vi "Load from History File.vi"(8 "error in (no error)":errorcluster, 11 "Data Manager in":refnum<class "Data Manager.lvclass">) -> (0 "error out":errorcluster, 2 "History":T1={"Record Headers"=["Athlete", "Team", "Type", "Date", "Distance", "Moving Time", "Elapsed Time", "Total Elevation Gain"], "All Records"=[]}, 3 "Data Manager out":refnum<class "Data Manager.lvclass">)   [LabVIEW 2020, in "Data Manager.lvclass"]
uses:
  Data Manager.lvclass
  Data Manager.lvclass/Data Manager.ctl
  Name--cluster.ctl
  Profile--cluster.ctl
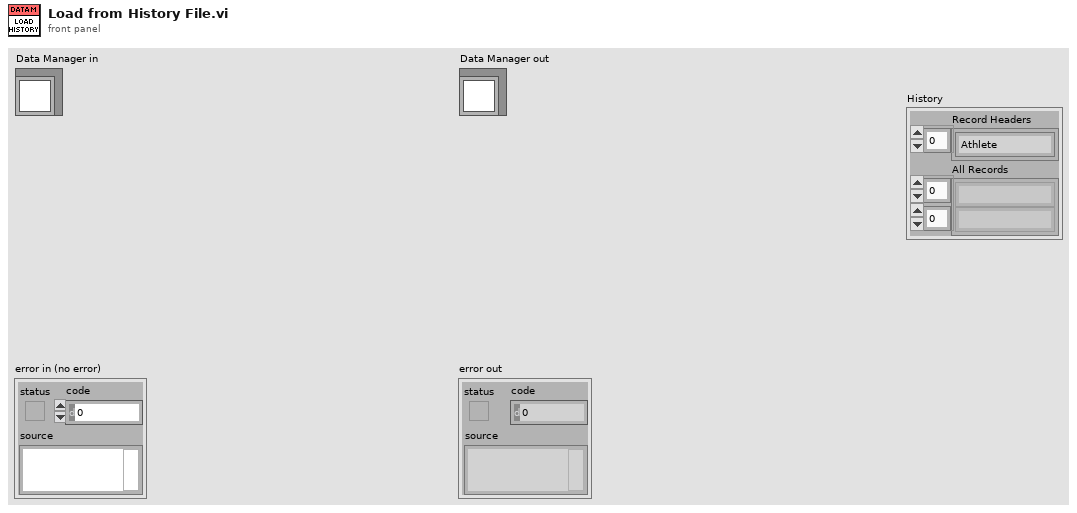
[diagram p1: front panel]
types:
  T1 = cluster{"Record Headers":string[], "All Records":string[][]}
  T2 = enum16{"open", "open or create", "create or replace", "create", "open (read-only)"}
  T3 = typedef "Data Manager.lvclass/Profile--cluster.ctl" = cluster{"Alias":string, "Team":string}
  T4 = typedef "Data Manager.lvclass/Name--cluster.ctl" = cluster{"First":string, "Last":string}
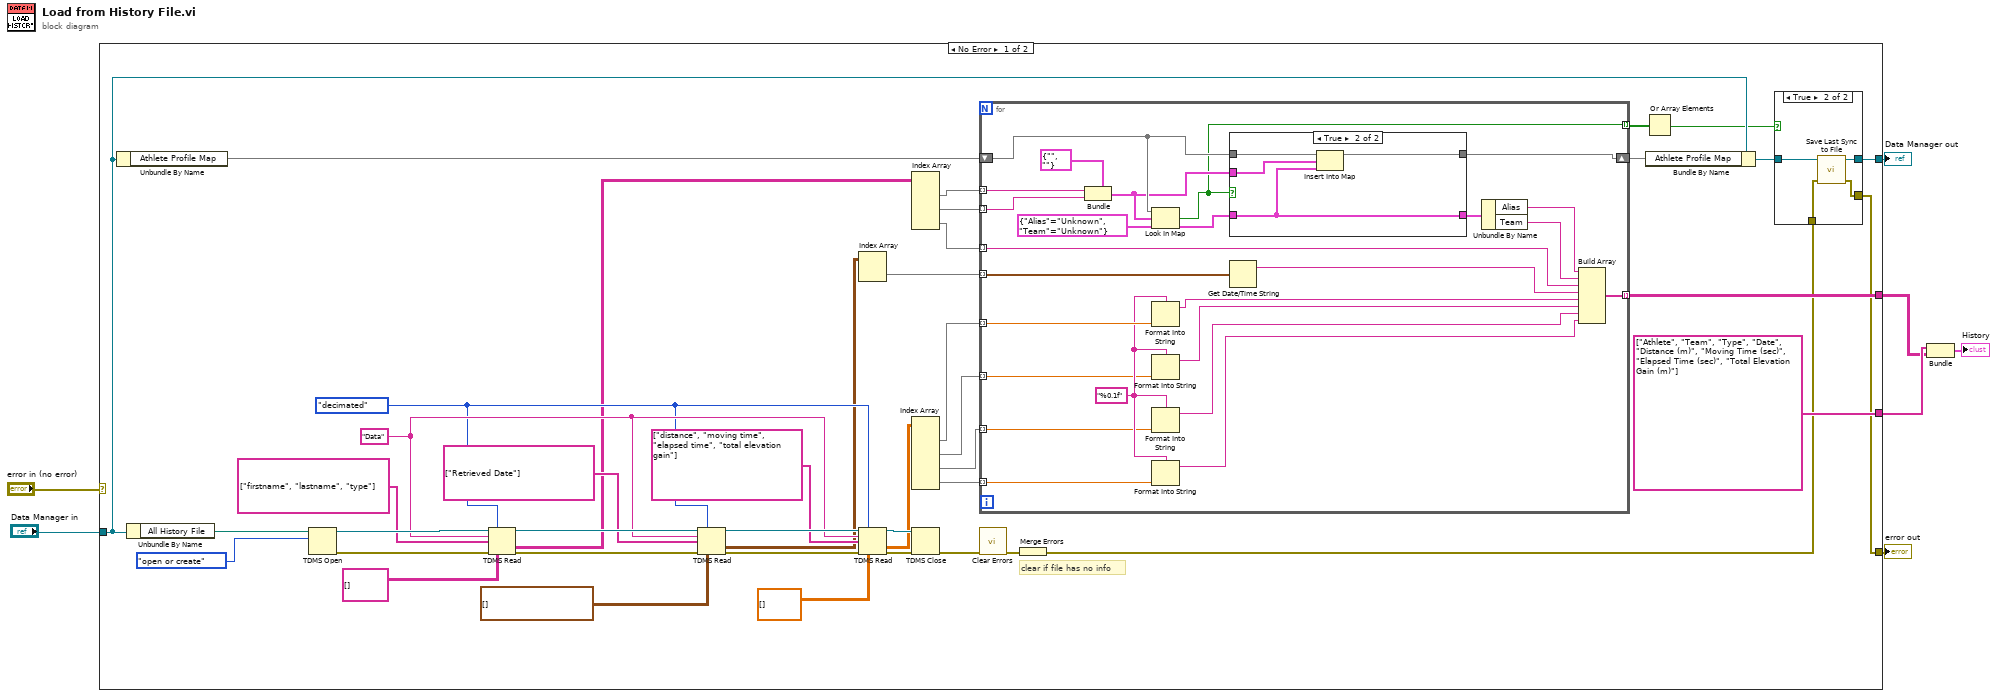
[diagram p0: block diagram]
diagram:
  n1 = case shown="No Error" "error in (no error)" {
    selector: "error in (no error)" -> [_ w88]
    tunnel: [w11 w88] -> w6
    tunnel: [w9 w87] -> w4
    tunnel: "Data Manager in" -> [w24 w87]
    tunnel: [string[] ["Athlete", "Team", "Type", "Date", "Distance (m)", "Moving Time (sec)", "Elapsed Time (sec)", "Total Elevation Gain (m)"] ("appended array") _] -> w3
    tunnel: [w15 _] -> w2
    frame No Error {
      w41 = enum16{"decimated", "interleaved"}."decimated" ("data layout (0:decimated)")
      w42 = "Data" ("group name in (Untitled)")
      # "clear if file has no info"
      n2 = Unbundle By Name(w24) -> ("Athlete Profile Map"=w26:map{T4, T3})
      n3 = Unbundle By Name(w24) -> ("All History File"=w40:path)
      n4 = TDMS Open(10:T2."open or create" ("operation (0:open)"), 11:w40) -> (0:w31:errorcluster, 3:w48:refnum<k34>)  [unwired: 5 in]
      n5 = TDMS Read(0:w48, 1:w41, 5:w42, 7:string[] ["firstname", "lastname", "type"] ("channel name(s) in (Untitled)"), 11:w31, 12:string[][] [] ("transposed array")) -> (4:w44:refnum<k34>, 10:w29:string[][], 15:w33:errorcluster)  [unwired: 2 in, 3 out]
      n6 = TDMS Read(0:w44, 1:w41, 5:w42, 7:string[] ["Retrieved Date"] ("channel name(s) in (Untitled)"), 11:w33, 12:timestamp[][] [] ("transposed array")) -> (4:w43:refnum<k34>, 10:w23:timestamp[][], 15:w32:errorcluster)  [unwired: 2 in, 3 out]
      n7 = Index Array(array=w23) -> (element=w22:timestamp[])  [unwired: 2 in]
      n8 = TDMS Read(0:w43, 1:w41, 5:w42, 7:string[] ["distance", "moving time", "elapsed time", "total elevation gain"] ("channel name(s) in (Untitled)"), 11:w32, 12:dbl[][] [] ("transposed array")) -> (4:w47:refnum<k34>, 10:w21:dbl[][], 15:w46:errorcluster)  [unwired: 2 in, 3 out]
      n9 = Index Array(array=w29) -> (element #1=w28:string[], element #2=w27:string[], element #3=w25:string[])  [unwired: 6 in]
      n10 = Index Array(array=w21) -> (element #1=w20:dbl[], element #2=w19:dbl[], element #3=w18:dbl[], element #4=w17:dbl[])  [unwired: 8 in]
      n11 = TDMS Close(8:w46, 11:w47) -> (0:w45:errorcluster)  [unwired: 1 out]
      n12 = for {
        tunnel: w28 -> [w79] mode=indexing
        tunnel: w27 -> [w78] mode=indexing
        shift-right: [w75] -> w14
        shift-left: w26 -> [w76]
        tunnel: w25 -> [w66] mode=indexing
        tunnel: w22 -> [w69] mode=indexing
        tunnel: w20 -> [w71] mode=indexing
        tunnel: w19 -> [w63] mode=indexing
        tunnel: w18 -> [w60] mode=indexing
        tunnel: w17 -> [w59] mode=indexing
        tunnel: [w57] -> w15 mode=indexing
        tunnel: [w56] -> w13 mode=indexing
        w70 = "%0.1f" ("format string")
        n13 = Bundle(cluster=T4 {"First"="", "Last"=""} ("Name"), "First"=w79, "Last"=w78) -> (w73:T4)
        n14 = Look In Map(map=w76, key=w73, default value=T3 {"Alias"="Unknown", "Team"="Unknown"}) -> (key not found?=w56:bool, value=w74:T3)
        n15 = Format Into String(format string=w70, w71) -> (resulting string=w64:string)  [unwired: 2 in, 1 out]
        n16 = Format Into String(format string=w70, w63) -> (resulting string=w62:string)  [unwired: 2 in, 1 out]
        n17 = Format Into String(format string=w70, w60) -> (resulting string=w61:string)  [unwired: 2 in, 1 out]
        n18 = Format Into String(format string=w70, w59) -> (resulting string=w58:string)  [unwired: 2 in, 1 out]
        n19 = case shown="True" w56 {
          tunnel: w76 -> [w82 w86]
          tunnel: [w82 w85] -> w75
          tunnel: w74 -> [w81 w83]
          tunnel: w73 -> [_ w84]
          tunnel: [w81 w83] -> w72
          frame False {
          }
          frame True {
            n20 = Insert Into Map(map in=w86, key=w84, value=w83) -> (map out=w85:map{T4, T3})  [unwired: 2 out]
          }
        }
        n21 = Get Date/Time String(seconds (now)=w69) -> (date string=w65:string)  [unwired: 2 in, 1 out]
        n22 = Unbundle By Name(w72) -> ("Alias"=w68:string, "Team"=w67:string)
        n23 = Build Array(w68, w67, w66, w65, w64, w62, w61, w58) -> (w57:string[])
      }
      n24 = call <vilib>:"Clear Errors.vi"("error in (no error)"=w45) -> ("error out"=w30:errorcluster)  [unwired: 5 in, 1 out]
      n25 = Merge Errors(w30) -> (w12:errorcluster)
      n26 = Bundle By Name(cluster=w24, "Athlete Profile Map"=w14) -> (w10:refnum<class "Data Manager.lvclass">)
      n27 = Or Array Elements(Boolean array=w13) -> (logical OR=w8:bool)
      n28 = case shown="True" w8 {
        tunnel: w12 -> [w50 w52]
        tunnel: [w50 w53] -> w11
        tunnel: w10 -> [w51 w55]
        tunnel: [w51 w54] -> w9
        frame False {
        }
        frame True {
          n29 = call-dynamic "Save Last Sync to File.vi"("error in (no error)"=w52, "Data Manager in"=w55) -> ("error out"=w53:errorcluster, "Data Manager out"=w54:refnum<class "Data Manager.lvclass">)  [unwired: 8 in]
        }
      }
    }
    frame Error {
    }
  }
  "error out" <- w6
  "Data Manager out" <- w4
  n30 = Bundle("appended array"=w3, w2) -> (→"History":cluster{"appended array":string[], string[][]})  [unwired: 1 in]
